vi "Update HWI.vi"(3 "Error In":errorcluster, 4 "Current Variables":T1[](array[typedef]), 6 "Devices queue":refnum<queue>) -> (0 "Error Out":errorcluster, 1 "Total Time":dbl, 2 "Devices queue out":refnum<queue>)   [LabVIEW 2013]
uses:
  TypeDefs/Active procedure variables.ctl
  Device/Device.lvclass
  Master Device/Master Device.lvclass
  PackedLibraries/LuaEvaluatorAPI.lvlibp/API/t_Caching_Expression_Evaluator_Methods_Table.ctl
  Globals/Total Time.vi
  PackedLibraries/LuaEvaluatorAPI.lvlibp
panel:
  out "Check HWI Timing":u32[](array[numeric])
  out "Finalize HWI Timing":u32[](array[numeric])
  out "Prep HWI Timing":u32[](array[numeric])
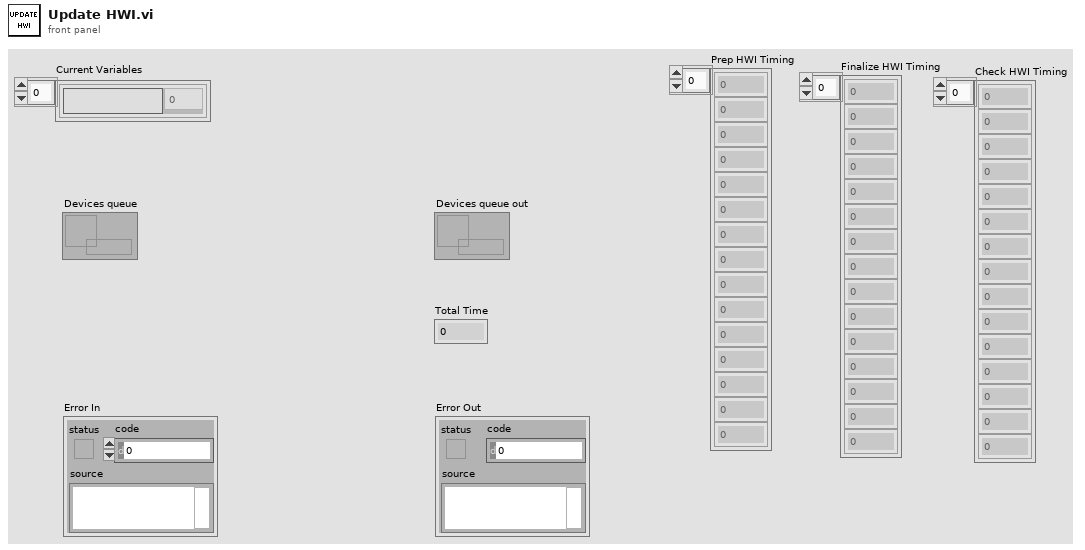
[diagram p1: front panel]
types:
  T1 = typedef "Active procedure variables.ctl" = cluster{"Procedure variable":string, "Value":dbl}
  T2 = typedef "LuaEvaluatorAPI.lvlibp/t_Caching_Expression_Evaluator_Methods_Table.ctl" = enum16{"set", "get", "eval", "assign", "isvalid", "execute", "evaltable", "close"}
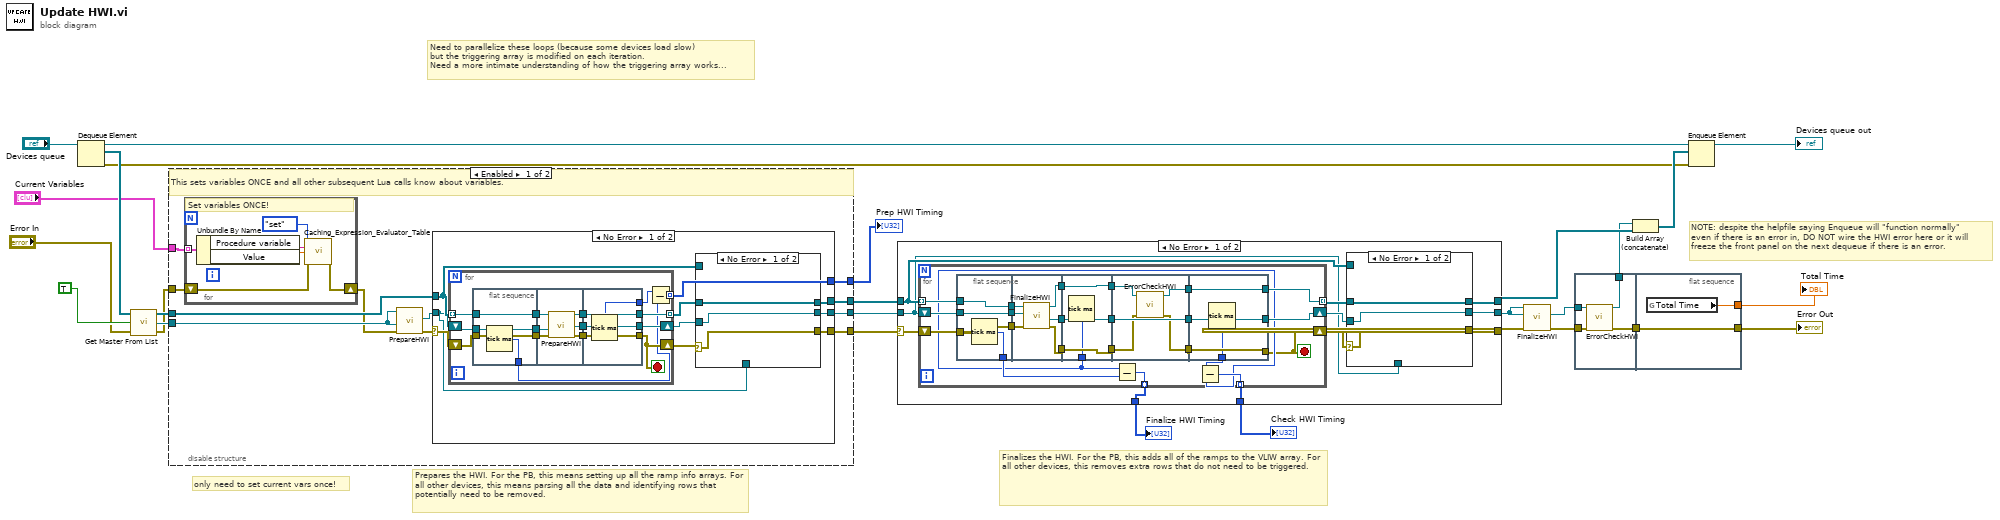
[diagram p0: block diagram]
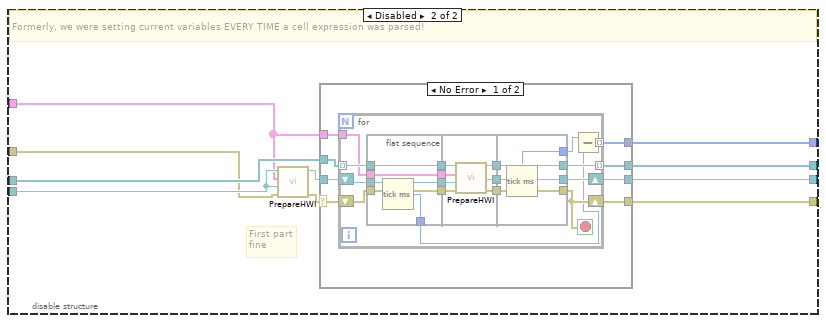
[diagram p4: hidden frame]
diagram:
  # "only need to set current vars once!"
  # "NOTE: despite the helpfile saying Enqueue will \"function normally\"\neven if there is an error in, DO NOT wire the HWI error here or it will\nfreeze the front panel on the next dequeue if there is an error."
  # "Finalizes the HWI. For the PB, this adds all of the ramps to the VLIW array. For all other devices, this removes extra rows that do not need to be triggered."
  # "Prepares the HWI. For the PB, this means setting up all the ramp info arrays. For all other devices, this means parsing all the data and identifying rows that potentially need to be removed."
  # "Need to parallelize these loops (because some devices load slow)\nbut the triggering array is modified on each iteration.\nNeed a more intimate understanding of how the triggering array works..."
  n1 = Dequeue Element(queue="Devices queue") -> (queue out=w8:refnum<queue>, element=w11:refnum<class "Device.lvclass">[], error out=w5:errorcluster)  [unwired: 2 in, 1 out]
  n2 = call "Get Master From List.vi"("error in"="Error In", "Del From List?"=TRUE, "Device List in"=w11) -> ("error out"=w3:errorcluster, "Master Device"=w22:refnum<class "Master Device.lvclass">, "Device List out"=w24:refnum<class "Device.lvclass">[])
  n3 = disable-structure shown="Enabled" {
    disable-tunnel: [w38 w102] -> w27
    disable-tunnel: [w37 w101] -> w26
    disable-tunnel: w24 -> [w36 w100]
    disable-tunnel: w22 -> [w35 w99]
    disable-tunnel: [w34 w97] -> w21
    disable-tunnel: [w33 w96] -> w15
    disable-tunnel: "Current Variables" -> [w29 w93]
    disable-tunnel: w3 -> [w31 w94]
    frame Enabled {
      # "This sets variables ONCE and all other subsequent Lua calls know about variables."
      n4 = for {
        shift-right: [w44] -> w30
        shift-left: w31 -> [w43]
        tunnel: w29 -> [w42] mode=indexing
        # "Set variables ONCE!"
        n5 = Unbundle By Name(w42) -> ("Procedure variable"=w41:string, "Value"=w40:dbl)
        n6 = call "Caching_Expression_Evaluator_Table.vi"("method"=t_Caching_Expression_Evaluator_Methods_Table."set", "variable"=w41, "value in"=w40, "error in (no error)"=w43) -> ("error out"=w44:errorcluster)  [unwired: 9 in, 2 out]
      }
      n7 = call-dynamic "PrepareHWI.vi"("error in (no error)"=w30, 9:"Master Device in"=w35, 11:"Master Device in"=w35) -> ("error out"=w32:errorcluster, "Master Device out"=w28:refnum<class "Master Device.lvclass">)  [unwired: 6 in, 1 out]
      n8 = case shown="No Error" w32 {
        selector: w32 -> [w54 w92]
        tunnel: [w51 w92] -> w38
        tunnel: [w47 w91] -> w37
        tunnel: w36 -> [w46 w91]
        tunnel: w28 -> [w45 w90]
        tunnel: [w49 w90] -> w34
        tunnel: [w53 _] -> w33
        frame No Error {
          n9 = for {
            shift-right: [w72] -> w52
            shift-left: w54 -> [w73]
            shift-right: [w71] -> w50
            shift-left: w45 -> [w74]
            tunnel: w46 -> [w75] mode=indexing
            tunnel: [w70] -> w48 mode=indexing
            tunnel: [w61] -> w53 mode=indexing
            stop <- w72 stop-if-true
            n10 = flat-sequence {
              tunnel: w73 -> [w77]
              tunnel: w74 -> [w78]
              tunnel: w75 -> [w79]
              tunnel: [w79] -> w69
              tunnel: [w78] -> w68
              tunnel: [w77] -> w67
              tunnel: [w76] -> w62
              tunnel: w69 -> [w85]
              tunnel: w68 -> [w84]
              tunnel: w67 -> [w83]
              tunnel: [w82] -> w66
              tunnel: [w81] -> w65
              tunnel: [w80] -> w64
              tunnel: [w87] -> w70
              tunnel: [w88] -> w71
              tunnel: [w89] -> w72
              tunnel: w66 -> [w89]
              tunnel: w65 -> [w88]
              tunnel: w64 -> [w87]
              tunnel: [w86] -> w63
              frame #0 {
                n11 = Tick Count (ms)() -> (millisecond timer value=w76:u32)
              }
              frame #1 {
                n12 = call-dynamic "PrepareHWI.vi"("error in (no error)"=w83, "Master Device in"=w84, "Device in"=w85) -> ("error out"=w82:errorcluster, "Master Device out"=w81:refnum<class "Master Device.lvclass">, "Device out"=w80:refnum<class "Device.lvclass">)  [unwired: 6 in]
              }
              frame #2 {
                n13 = Tick Count (ms)() -> (millisecond timer value=w86:u32)
              }
            }
            n14 = Subtract(x=w63, y=w62) -> (x-y=w61:u32)
          }
          n15 = case shown="No Error" w52 {
            selector: w52 -> [w57 w58]
            tunnel: [w57 w58] -> w51
            tunnel: w50 -> [w56 _]
            tunnel: [w56 w59] -> w49
            tunnel: w48 -> [w55 _]
            tunnel: [w55 w60] -> w47
            tunnel: w46 -> [_ w60]
            tunnel: w45 -> [_ w59]
            frame No Error {
            }
            frame Error {
              # "Keep unmodified devices if there is an error"
            }
          }
        }
        frame Error {
        }
      }
    }
    frame Disabled {
      # "First part\nfine"
      # "Formerly, we were setting current variables EVERY TIME a cell expression was parsed!"
      n16 = call-dynamic "PrepareHWI.vi"("error in (no error)"=w94, 9:"Master Device in"=w99, "Current Variables"=w93, 11:"Master Device in"=w99) -> ("error out"=w95:errorcluster, "Master Device out"=w98:refnum<class "Master Device.lvclass">)  [unwired: 5 in, 1 out]
      n17 = case shown="No Error" w95 {
        selector: w95 -> [w110 w146]
        tunnel: [w105 w146] -> w102
        tunnel: [w106 w145] -> w101
        tunnel: w100 -> [w107 w145]
        tunnel: w98 -> [w109 w144]
        tunnel: w93 -> [w108 _]
        tunnel: [w104 w144] -> w97
        tunnel: [w103 _] -> w96
        frame No Error {
          n18 = for {
            shift-right: [w123] -> w105
            shift-left: w110 -> [w124]
            shift-right: [w122] -> w104
            shift-left: w109 -> [w125]
            tunnel: w108 -> [w126]
            tunnel: w107 -> [w127] mode=indexing
            tunnel: [w121] -> w106 mode=indexing
            tunnel: [w111] -> w103 mode=indexing
            stop <- w123 stop-if-true
            n19 = flat-sequence {
              tunnel: w124 -> [w129]
              tunnel: w125 -> [w130]
              tunnel: w126 -> [w131]
              tunnel: w127 -> [w132]
              tunnel: [w132] -> w120
              tunnel: [w131] -> w119
              tunnel: [w130] -> w118
              tunnel: [w129] -> w117
              tunnel: [w128] -> w112
              tunnel: w120 -> [w139]
              tunnel: w119 -> [w138]
              tunnel: w118 -> [w137]
              tunnel: w117 -> [w136]
              tunnel: [w135] -> w116
              tunnel: [w134] -> w115
              tunnel: [w133] -> w114
              tunnel: [w141] -> w121
              tunnel: [w142] -> w122
              tunnel: [w143] -> w123
              tunnel: w116 -> [w143]
              tunnel: w115 -> [w142]
              tunnel: w114 -> [w141]
              tunnel: [w140] -> w113
              frame #0 {
                n20 = Tick Count (ms)() -> (millisecond timer value=w128:u32)
              }
              frame #1 {
                n21 = call-dynamic "PrepareHWI.vi"("error in (no error)"=w136, "Master Device in"=w137, "Current Variables"=w138, "Device in"=w139) -> ("error out"=w135:errorcluster, "Master Device out"=w134:refnum<class "Master Device.lvclass">, "Device out"=w133:refnum<class "Device.lvclass">)  [unwired: 5 in]
              }
              frame #2 {
                n22 = Tick Count (ms)() -> (millisecond timer value=w140:u32)
              }
            }
            n23 = Subtract(x=w113, y=w112) -> (x-y=w111:u32)
          }
        }
        frame Error {
        }
      }
    }
  }
  "Prep HWI Timing" <- w15
  n24 = case shown="No Error" w27 {
    selector: w27 -> [w157 w212]
    tunnel: [w152 w212] -> w20
    tunnel: w26 -> [w148 w211]
    tunnel: [w153 w211] -> w25
    tunnel: w21 -> [w147 w210]
    tunnel: [w154 w210] -> w19
    tunnel: [w156 _] -> w14
    tunnel: [w155 _] -> w13
    frame No Error {
      n25 = for {
        shift-right: [w164] -> w151
        shift-left: w157 -> [w184]
        shift-right: [w176] -> w150
        shift-left: w147 -> [w185]
        tunnel: w148 -> [w186] mode=indexing
        tunnel: [w177] -> w149 mode=indexing
        tunnel: [w168] -> w156 mode=indexing
        tunnel: [w167] -> w155 mode=indexing
        stop <- w164 stop-if-true
        n26 = flat-sequence {
          tunnel: w184 -> [w188]
          tunnel: w185 -> [w189]
          tunnel: w186 -> [w190]
          tunnel: [w190] -> w172
          tunnel: [w189] -> w171
          tunnel: [w188] -> w170
          tunnel: [w187] -> w169
          tunnel: [w193] -> w183
          tunnel: [w192] -> w182
          tunnel: [w191] -> w181
          tunnel: w172 -> [w196]
          tunnel: w171 -> [w195]
          tunnel: w170 -> [w194]
          tunnel: w183 -> [w200]
          tunnel: w182 -> [w199]
          tunnel: w181 -> [w198]
          tunnel: [w200] -> w180
          tunnel: [w199] -> w179
          tunnel: [w198] -> w178
          tunnel: [w197] -> w165
          tunnel: w180 -> [w203]
          tunnel: w179 -> [w205]
          tunnel: w178 -> [w202]
          tunnel: [w201] -> w175
          tunnel: [w204] -> w174
          tunnel: [w203] -> w173
          tunnel: [w207] -> w176
          tunnel: [w208] -> w177
          tunnel: [w209] -> w164
          tunnel: w175 -> [w209]
          tunnel: w174 -> [w208]
          tunnel: w173 -> [w207]
          tunnel: [w206] -> w166
          frame #0 {
            n27 = Tick Count (ms)() -> (millisecond timer value=w187:u32)
          }
          frame #1 {
            n28 = call-dynamic "FinalizeHWI.vi"("error in (no error)"=w194, "Master Device in"=w195, "Device in"=w196) -> ("error out"=w191:errorcluster, "Master Device out"=w193:refnum<class "Master Device.lvclass">, "Device out"=w192:refnum<class "Device.lvclass">)  [unwired: 6 in]
          }
          frame #2 {
            n29 = Tick Count (ms)() -> (millisecond timer value=w197:u32)
          }
          frame #3 {
            n30 = call-dynamic "ErrorCheckHWI.vi"("error in (no error)"=w202, "Device in"=w205) -> ("error out"=w201:errorcluster, "Device out"=w204:refnum<class "Device.lvclass">)  [unwired: 8 in]
          }
          frame #4 {
            n31 = Tick Count (ms)() -> (millisecond timer value=w206:u32)
          }
        }
        n32 = Subtract(x=w165, y=w169) -> (x-y=w168:u32)
        n33 = Subtract(x=w166, y=w165) -> (x-y=w167:u32)
      }
      n34 = case shown="No Error" w151 {
        selector: w151 -> [w160 w161]
        tunnel: [w160 w161] -> w152
        tunnel: w150 -> [w159 _]
        tunnel: [w159 w162] -> w154
        tunnel: w149 -> [w158 _]
        tunnel: [w158 w163] -> w153
        tunnel: w148 -> [_ w163]
        tunnel: w147 -> [_ w162]
        frame No Error {
        }
        frame Error {
          # "Keep unmodified devices if there is an error"
        }
      }
    }
    frame Error {
    }
  }
  "Finalize HWI Timing" <- w14
  "Check HWI Timing" <- w13
  n35 = call-dynamic "FinalizeHWI.vi"("error in (no error)"=w20, 10:"Master Device in"=w19, 11:"Master Device in"=w19) -> ("error out"=w17:errorcluster, "Master Device out"=w18:refnum<class "Master Device.lvclass">)  [unwired: 6 in, 1 out]
  n36 = flat-sequence {
    tunnel: w18 -> [w216]
    tunnel: w17 -> [w215]
    tunnel: [w214] -> w16
    tunnel: [w213] -> w2
    tunnel: [w218] -> w7
    tunnel: w2 -> [w218]
    tunnel: [w217] -> w1
    frame #0 {
      n37 = call-dynamic "ErrorCheckHWI.vi"("error in (no error)"=w215, "Device in"=w216) -> ("error out"=w213:errorcluster, "Device out"=w214:refnum<class "Master Device.lvclass">)  [unwired: 8 in]
    }
    frame #1 {
      n38 = global read "Total Time.vi" "Total Time"() -> (w217:dbl)
    }
  }
  n39 = Build Array (concatenate)(w16, w25) -> (w10:refnum<class "Device.lvclass">[])
  n40 = Enqueue Element(queue=w8, element=w10, error in (no error)=w5) -> (queue out=→"Devices queue out":refnum<queue>)  [unwired: 1 in, 2 out]
  "Error Out" <- w7
  "Total Time" <- w1
